vi "Digital Bank Read.vi"(8 "error in (no error)":errorcluster, 11 "TCP Network Connection in":refnum<k5>) -> (0 "error out":errorcluster, 2 "States":i16[](array[numeric]), 3 "TCP Network Connection out":refnum<k5>)   [LabVIEW 2024, in "OptoMMP.lvlib"]
doc: "Performs a digital bank read on the specified TCP network and returns an array of 64 channel states. NaN is written to channels if a communication error occurs.\n\nIn order from top to bottom, the \"States\" array corresponds to channel 0 of module 0 through channel 4 of module 15 (increasing order). \"Digital Bank Read\" must be preceded by \"OptoMMP Open Connection\" or \"Powerup Clear\" if a new connection has been established.\n\nLast updated: 8/6/2025"
uses:
  <instrlib>/OptoMMP/OptoMMP.lvlib
panel:
  # "Copyright (c) 2025 California Institute of Technology (Caltech).\nU.S. Government sponsorship acknowledged.\n\nLicensed under the Apache License, Version 2.0 (the \"License\");\nyou may not use this file except in compliance with the License.\nYou may obtain a copy of the License at\n\n    http://www.apache.org/licenses/LICENSE-2.0\n\nUnless required by applicable law or agreed to in writing, software\ndistributed under the License is distributed on an \"AS IS\" BASIS,\nWITHOUT WARRANTIES OR CONDITIONS OF ANY KIND, either express or implied.\nSee the License for the specific language governing permissions and\nlimitations under the License."
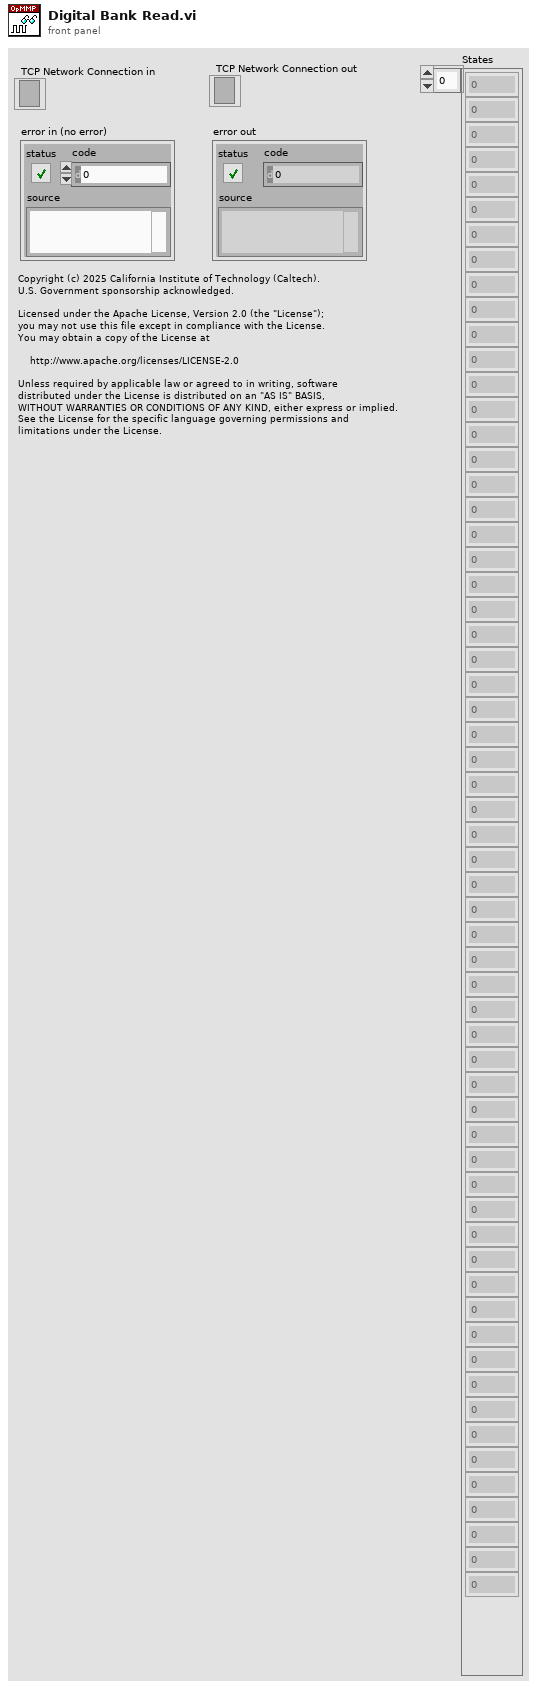
[diagram p1: front panel]
types:
  T1 = enum16{"Read Block Response", "Write Quadlet or Block Response", "Read Quadlet Response"}
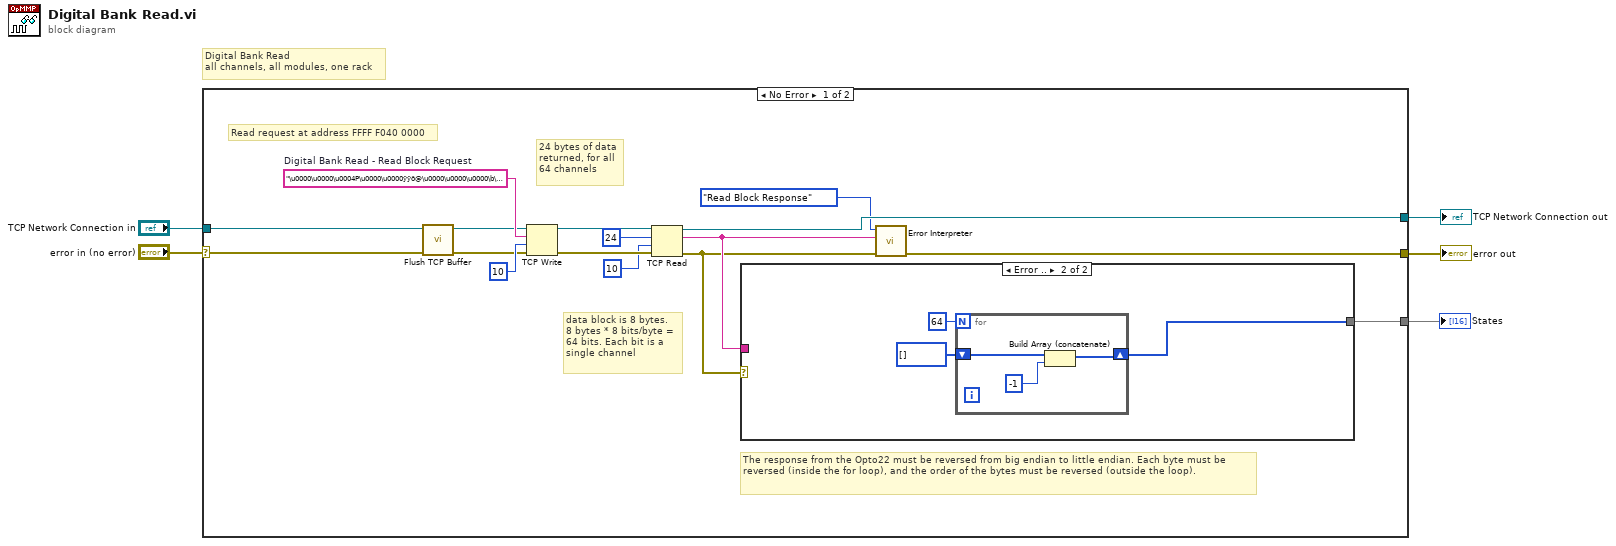
[diagram p0: block diagram]
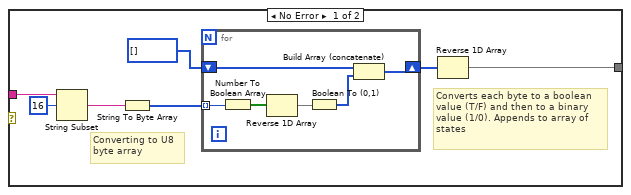
[diagram p2: hidden frame]
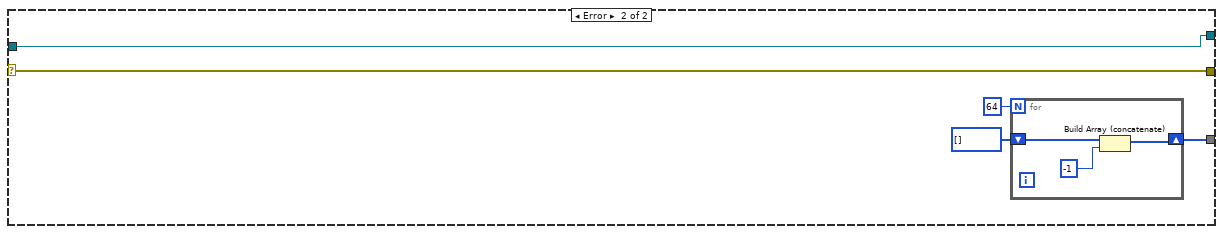
[diagram p3: hidden frame]
diagram:
  # "Digital Bank Read\nall channels, all modules, one rack"
  n1 = case shown="No Error" "error in (no error)" {
    selector: "error in (no error)" -> [w8 w41]
    tunnel: [w21 w45] -> w5
    tunnel: [w20 w41] -> w4
    tunnel: "TCP Network Connection in" -> [w9 w45]
    tunnel: [w19 w42] -> w2
    frame No Error {
      w18 = "\u0000\u0000\u0004P\u0000\u0000ÿÿð@\u0000\u0000\u0000\b\u0000\u0000"  # Digital Bank Read - Read Block Request
      # "Read request at address FFFF F040 0000"
      # "data block is 8 bytes.\n8 bytes * 8 bits/byte =\n64 bits. Each bit is a \nsingle channel"
      # "24 bytes of data\nreturned, for all\n64 channels"
      # "The response from the Opto22 must be reversed from big endian to little endian. Each byte must be reversed (inside the for loop), and the order of the bytes must be reversed (outside the loop)."
      n2 = call <instrlib>:"Flush TCP Buffer.vi"("error in (no error)"=w8, "TCP Network Connection in"=w9) -> ("error out"=w6:errorcluster, "TCP Network Connection out"=w7:refnum<k5>)  [unwired: 8 in]
      n3 = TCP Write(connection ID=w7, data in=w18, error in (no error)=w6, 9:10 ("timeout ms (25000)")) -> (connection ID out=w16:refnum<k5>, error out=w15:errorcluster)  [unwired: 1 out]
      n4 = TCP Read(connection ID=w16, bytes to read=24, error in (no error)=w15, 9:10 ("timeout ms (25000)")) -> (connection ID out=w21:refnum<k5>, data out=w12:string, error out=w11:errorcluster)  [unwired: 1 in]
      n5 = case shown="Error .." w11 {
        tunnel: w12 -> [w23 _]
        tunnel: [w22 w36] -> w19
        frame No Error {
          # "Converts each byte to a boolean\nvalue (T/F) and then to a binary\nvalue (1/0). Appends to array of\nstates"
          # "Converting to U8\nbyte array"
          n6 = String Subset(string=w23, offset (0)=16) -> (substring=w26:string)  [unwired: 1 in]
          n7 = String To Byte Array(string=w26) -> (unsigned byte array=w27:u8[])
          n8 = for {
            tunnel: w27 -> [w34] mode=indexing
            shift-right: [w32] -> w24
            shift-left: i16[] [] -> [w31]
            n9 = Number To Boolean Array(number=w34) -> (Boolean array=w30:bool[])
            n10 = Reverse 1D Array(array=w30) -> (reversed array=w29:bool[])
            n11 = Boolean To (0,1)(Boolean=w29) -> (0, 1=w33:i16[])
            n12 = Build Array (concatenate)(w31, w33) -> (w32:i16[])
          }
          n13 = Reverse 1D Array(array=w24) -> (reversed array=w22:i16[])
        }
        frame Error {
          n14 = for {
            N: 64 -> [_]
            shift-right: [w39] -> w36
            shift-left: i16[] [] -> [w38]
            n15 = Build Array (concatenate)(w38, i16 -1) -> (w39:i16[])
          }
        }
      }
      n16 = call <instrlib>:"Error Interpreter.vi"("error in (no error)"=w11, "data in"=w12, "packet type"=T1."Read Block Response") -> ("error out"=w20:errorcluster)  [unwired: 8 in]
    }
    frame Error {
      n17 = for {
        N: 64 -> [_]
        shift-right: [w47] -> w42
        shift-left: i16[] [] -> [w46]
        n18 = Build Array (concatenate)(w46, i16 -1) -> (w47:i16[])
      }
    }
  }
  "TCP Network Connection out" <- w5
  "error out" <- w4
  "States" <- w2
